vi "Get String.vi"(8 "error in":errorcluster, 10 "CMD":string="R1", 11 "handle in":T1) -> (0 "error out":errorcluster, 2 "DataOut":string, 3 "handle out":T1)   [LabVIEW 2015, in "Text Device Session.lvclass"]
doc: "Retrieve a string from the port - no conversion required."
uses:
  Text Communication/Text Device Session.lvclass
  <userlib>/_Session Fwk/Typedefs/Session Handle.ctl
  <userlib>/_Session Fwk/Session - Root.lvclass
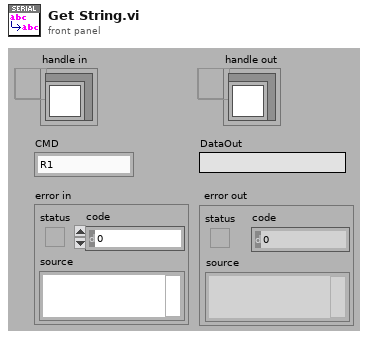
[diagram p1: front panel]
types:
  T1 = typedef "Session - Root.lvclass/Session Handle.ctl" = refnum<data-value>
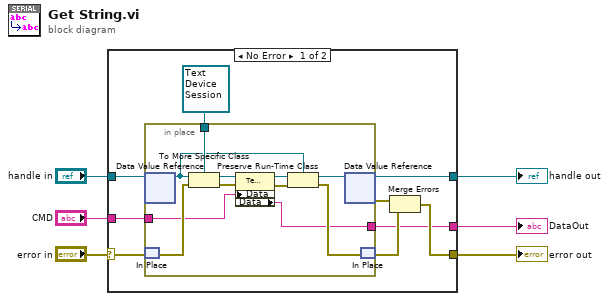
[diagram p0: block diagram]
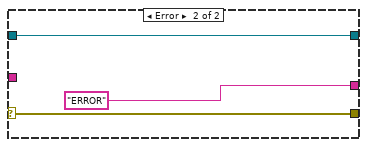
[diagram p2: hidden frame]
diagram:
  n1 = case shown="No Error" "error in" {
    selector: "error in" -> [w10 w28]
    tunnel: "handle in" -> [w15 w29]
    tunnel: [w14 w29] -> w5
    tunnel: [w11 w28] -> w1
    tunnel: "CMD" -> [w9 _]
    tunnel: [w8 "ERROR" ("Data")] -> w2
    frame No Error {
      n2 = in-place {
        in-place-border: w9 -> [w22]
        in-place-border: [w16] -> w8
        in-place-border: refnum<class "Text Device Session.lvclass"> refnum ("Text Session") -> [w25]
        n3 = in-place-dvr #1(w15) -> (w20:refnum<class "Session - Root.lvclass">)  [unwired: 1 out]
        n4 = in-place-match #2(w10) -> (w26:errorcluster)
        n5 = To More Specific Class(target class=w25, reference=w20, error in=w26) -> (specific class reference=w24:refnum<class "Text Device Session.lvclass">, error out=w23:errorcluster)
        n6 = property class="Text Session"(reference=w24, error in=w23, "Data"=w22) -> (reference out=w21:refnum<class "Text Device Session.lvclass">, error out=w17:errorcluster, "Data"=w16:string)
        n7 = Preserve Run-Time Class(object in=w21, error in=w17, 2:w20) -> (object out=w19:refnum<class "Session - Root.lvclass">, error out=w18:errorcluster)
        n8 = in-place-dvr #1(w19) -> (w14:T1, w12:errorcluster)
        n9 = in-place-match #2(w18) -> (w13:errorcluster)
      }
      n10 = Merge Errors(w12, w13) -> (w11:errorcluster)
    }
    frame Error {
    }
  }
  "error out" <- w1
  "DataOut" <- w2
  "handle out" <- w5
